vi "Main.vi"() -> ()   [LabVIEW 2017, in "MementoPatternDemo.lvclass"]
uses:
  MementoPatternDemo.lvclass
  Originator Class/Originator.lvclass
  CareTaker Class/CareTaker.lvclass
  Memento Class/Memento.lvclass
  ConsoleOut/Print Options.ctl
  Originator Class/Originator.lvclass/Originator.ctl
panel:
  out "error out":errorcluster
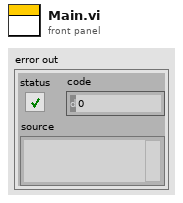
[diagram p1: front panel]
types:
  T1 = typedef "Print Options.ctl" = enum16{"Create", "Get Reference", "Print", "Print Header", "Close"}
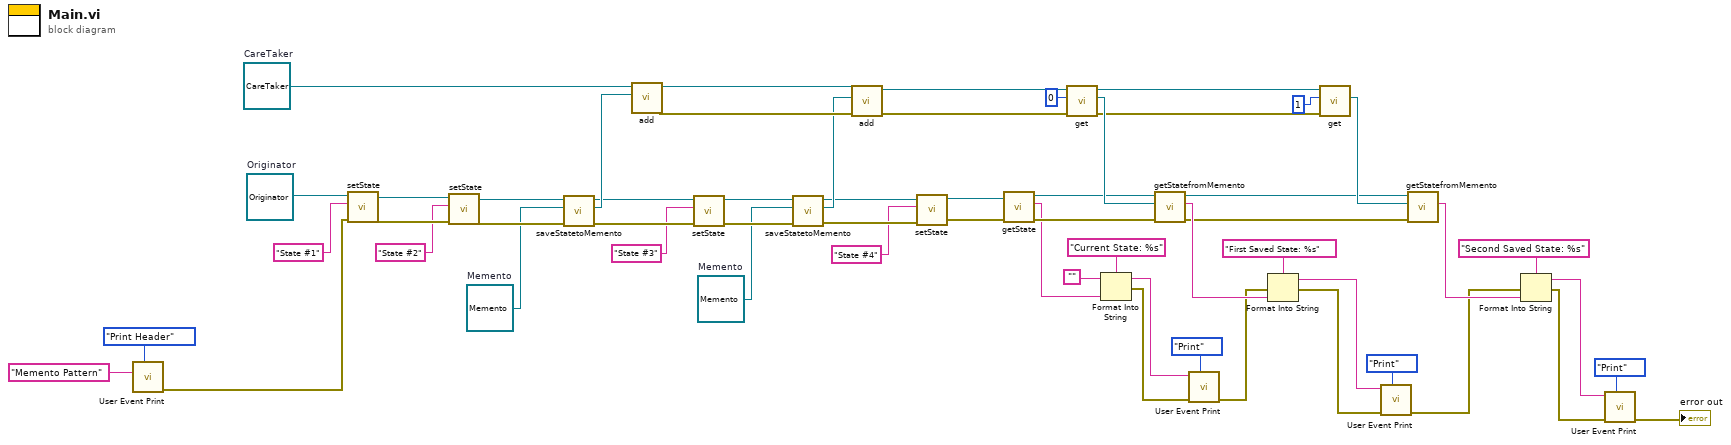
[diagram p0: block diagram]
diagram:
  w43 = refnum<class "Memento.lvclass"> refnum  # Memento
  w50 = refnum<class "CareTaker.lvclass"> refnum  # CareTaker
  w51 = refnum<class "Memento.lvclass"> refnum  # Memento
  w56 = refnum<class "Originator.lvclass"> refnum  # Originator
  n1 = call "User Event Print.vi"("Options"=Print_Options."Print Header", "String to Print"="Memento Pattern") -> ("error out"=w3:errorcluster)  [unwired: 8 in, 1 out]
  n2 = call "setState.vi"("error in (no error)"=w3, "State"="State #1", "Originator in"=w56) -> ("error out"=w57:errorcluster, "Originator out"=w58:refnum<class "Originator.lvclass">)  [unwired: 7 in]
  n3 = call "setState.vi"("error in (no error)"=w57, "State"="State #2", "Originator in"=w58) -> ("error out"=w52:errorcluster, "Originator out"=w53:refnum<class "Originator.lvclass">)  [unwired: 7 in]
  n4 = call "saveStatetoMemento.vi"("error in (no error)"=w52, "Memento In"=w51, "Originator in"=w53) -> ("error out"=w47:errorcluster, "Memento On"=w49:refnum<class "Memento.lvclass">, "Originator out"=w48:refnum<class "Originator.lvclass">)  [unwired: 6 in]
  n5 = call "add.vi"("Memento.lvclass"=w49, "CareTaker in"=w50) -> ("error out"=w41:errorcluster, "CareTaker out"=w42:refnum<class "CareTaker.lvclass">)  [unwired: 8 in]
  n6 = call "setState.vi"("error in (no error)"=w47, "State"="State #3", "Originator in"=w48) -> ("error out"=w44:errorcluster, "Originator out"=w45:refnum<class "Originator.lvclass">)  [unwired: 7 in]
  n7 = call "saveStatetoMemento.vi"("error in (no error)"=w44, "Memento In"=w43, "Originator in"=w45) -> ("error out"=w38:errorcluster, "Memento On"=w40:refnum<class "Memento.lvclass">, "Originator out"=w39:refnum<class "Originator.lvclass">)  [unwired: 6 in]
  n8 = call "add.vi"("error in (no error)"=w41, "Memento.lvclass"=w40, "CareTaker in"=w42) -> ("error out"=w35:errorcluster, "CareTaker out"=w36:refnum<class "CareTaker.lvclass">)  [unwired: 7 in]
  n9 = call "setState.vi"("error in (no error)"=w38, "State"="State #4", "Originator in"=w39) -> ("error out"=w33:errorcluster, "Originator out"=w22:refnum<class "Originator.lvclass">)  [unwired: 7 in]
  n10 = call "getState.vi"("error in (no error)"=w33, "Originator in"=w22) -> ("error out"=w23:errorcluster, "State"=w18:string, "Originator out"=w21:refnum<class "Originator.lvclass">)  [unwired: 7 in]
  n11 = call "get.vi"("error in (no error)"=w35, "index"=0, "CareTaker in"=w36) -> ("error out"=w15:errorcluster, "Memento.lvclass"=w32:refnum<class "Memento.lvclass">, "CareTaker out"=w14:refnum<class "CareTaker.lvclass">)  [unwired: 6 in]
  n12 = Format Into String(format string="Current State: %s", initial string="", w18) -> (resulting string=w12:string, error out=w17:errorcluster)  [unwired: 1 in]
  n13 = call "getStatefromMemento.vi"("error in (no error)"=w23, "Memento In"=w32, "Originator in"=w21) -> ("error out"=w24:errorcluster, "State"=w30:string, "Originator out"=w25:refnum<class "Originator.lvclass">)  [unwired: 6 in]
  n14 = call "User Event Print.vi"("Options"=Print_Options."Print", "error in (no error)"=w17, "String to Print"=w12) -> ("error out"=w13:errorcluster)  [unwired: 7 in, 1 out]
  n15 = Format Into String(format string="First Saved State: %s", error in=w13, w30) -> (resulting string=w9:string, error out=w16:errorcluster)  [unwired: 1 in]
  n16 = call "get.vi"("error in (no error)"=w15, "index"=1, "CareTaker in"=w14) -> ("Memento.lvclass"=w27:refnum<class "Memento.lvclass">)  [unwired: 6 in, 2 out]
  n17 = call "User Event Print.vi"("Options"=Print_Options."Print", "error in (no error)"=w16, "String to Print"=w9) -> ("error out"=w10:errorcluster)  [unwired: 7 in, 1 out]
  n18 = call "getStatefromMemento.vi"("error in (no error)"=w24, "Memento In"=w27, "Originator in"=w25) -> ("State"=w29:string)  [unwired: 6 in, 2 out]
  n19 = Format Into String(format string="Second Saved State: %s", error in=w10, w29) -> (resulting string=w7:string, error out=w6:errorcluster)  [unwired: 1 in]
  n20 = call "User Event Print.vi"("Options"=Print_Options."Print", "error in (no error)"=w6, "String to Print"=w7) -> ("error out"=→"error out":errorcluster)  [unwired: 7 in, 1 out]
